vi "pco.labview_Live_Example_COL.vi"() -> ()   [LabVIEW 2019]
doc: "A short program to demonstrate the fundamentals of control and image acquision with the pco.camera series. The program records a sequence of images, with \"live\" updating, until the \"StopRecording\" button is pressed. Use ctrl-H for more help on the individual controls and indicators.\n\nCopyright 2004, 2010 The Cooke Corporation."
uses:
  pco.sdk/CameraAccess/CameraAccess.lvlib
  pco.sdk/ImageSensor/ImageSensor.lvlib
  pco.sdk/TimingControl/TimingControl.lvlib
  pco.recorder/Recorder.lvlib
  pco.sdk/RecordingControl/RecordingControl.lvlib
  pco.sdk/CameraDescription/CameraDescription.lvlib
  pco.convert/Convert.lvlib
  pco.sdk/GeneralCameraControl/GeneralCameraControl.lvlib
  <vilib>/picture/picture.llb/Draw True-Color Pixmap.vi
panel:
  in  "Auto Range Crop":bool
  in  "Auto Range Peak":bool
  out "yHWOffset":u16
  out "xHWOffset":u16
  in  "iContrast [%]":i32 min=-100 max=100 step=1
  in  "Gamma":dbl=1.0 min=0.009999999776482582 max=10.0 step=0.009999999776482582 format="%.2f"
  out "wImgBuf":u16[][](array[numeric])
  in  "whiteBalance":bool
  in  "Zoom [%]":i32(slide)=26 min=10 max=200 step=5 scale=10.0..200.0
  in  "iScale_max":i32=60000 min=0 max=65535 step=1
  in  "iScale_min":i32=200 min=0 max=65535 step=1
  out "colorPattern":u16
  out "phConv":u64
  out "Image":picture
  out "Recorded Images":u32
  in  "TriggerMode":u16(ring) items=["auto sequence"=0, "software trigger"=1, "external exposure start & software trigger"=2, "external exposure control"=3, "external synchronized"=4, "fast external exposure control"=5, "external CDS control"=6, "slow external exposure control"=7, "external synchronized HDSDI"=258]
  in  "Quit":bool
  out "Error":errorcluster {"code" format="%x"}
  in  "Stop Record":bool
  out "Recording On":bool
  in  "roiY1":u16=2 min=2 max=1440 step=1
  in  "roiX1":u16=2 min=2 max=1920 step=1
  in  "roiY0":u16=1 min=1 max=1439 step=1
  in  "roiX0":u16=1 min=1 max=1919 step=1
  out "Image Height":u16
  out "Image Width":u16
  in  "Image Index":u32 max=9
  in  "dwImgCount":u32=10 caption="Required Number of Images" min=4 max=2247
  in  "DelayTimeBase":u16(ring)=2 items=["nanoseconds", "microseconds", "milliseconds"]
  in  "ExposureTimeBase":u16(ring)=2 items=["nanoseconds", "microseconds", "milliseconds"]
  in  "Exposure":u32=10 min=1
  in  "Delay":u32
  in  "Rate":i32(ring) items=["Low", "High"]
  # "This example is only suitable for color cameras\n\nThis example is similar to pco.labview_Live_Example.vi, but suited for color cameras.\nBecause n addition here also the convert library is used in order to get a truecolor image that is displayed\nWith the White Balance button it is possible to set the white balance, \nthe image value range can be selected with iScale_min/iScale_max, additionally contrast and gamma values can be selected\n\nUsage:\nSelect your required image count and the camera setup before you start the program.\nOnce started, the camera will be opened, the recorder will be created, initialized and images will be recorded and displayed automatically\nYou can stop the images by pressing stop record.\nAfter stopped, the image at the selected index will be read out\nTo finish the program click on quit application, this will force free and delete of the recorder and a close camera\nYou can change your required ROI, the value range, scaling, gamma, contrast  and the white balance after and also during record."
  # "pco.labview"
  # "Camera Setup"
  # "Recording Control"
  # "Parameters for image readout"
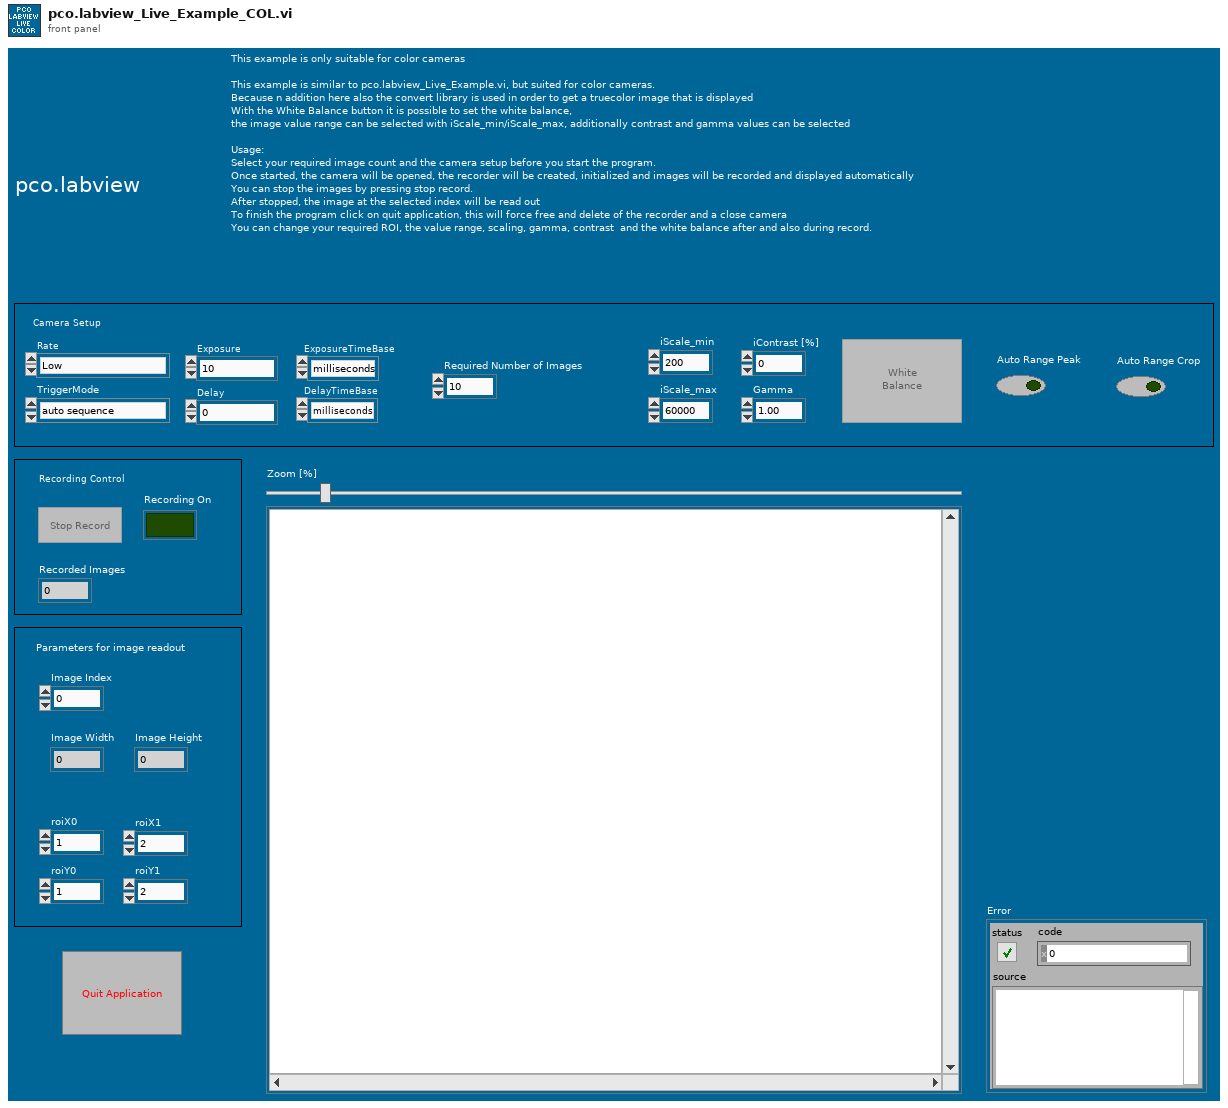
[diagram p1: front panel]
types:
  T1 = enum8{"Enabled", "Disabled", "Disabled and Grayed Out"}
  T2 = cluster{"wSensorTypeDESC":u16, "wSensorSubTypeDESC":u16, "wMaxHorzResStdDESC":u16, "wMaxVertResStdDESC":u16, "wMaxHorzResExtDESC":u16, "wMaxVertResExtDESC":u16, "wDynResDESC":u16, "wMaxBinHorzDESC":u16, "wBinHorzSteppingDESC":u16, "wMaxBinVertDESC":u16, "wBinVertSteppingDESC":u16, "wRoiHorStepsDESC":u16, "wRoiVertStepsDESC":u16, "wNumADCsDESC":u16, "wMinSizeHorzDESC":u16, "dwPixelRateDESC":u32[], "wConvFactDESC":u16[], "sCoolingSetpoints":i16[], "wSoftRoiHorStepsDESC":u16, "wSoftRoiVertStepsDESC":u16, "wIRDESC":u16, "wMinSizeVertDESC":u16, "dwMinDelayDESC":u32, "dwMaxDelayDESC":u32, "dwMinDelayStepDESC":u32, "dwMinExposureDESC":u32, "dwMaxExposureDESC":u32, "dwMinExposureStepDESC":u32, "dwMinDelayIRDESC":u32, "dwMaxDelayIRDESC":u32, "dwMinExposureIRDESC":u32, "dwMaxExposureIRDESC":u32, "wTimeTableDESC":u16, "wDoubleImageDESC":u16, "sMinCoolSetDESC":i16, "sMaxCoolSetDESC":i16, "sDefaultCoolSetDESC":i16, "wPowerDownModeDESC":u16, "wOffsetRegulationDESC":u16, "wColorPatternDESC":u16, "wPatternTypeDESC":u16, "wNumCoolingSetpoints":u16, "dwGeneralCapsDESC1":u32, "dwGeneralCapsDESC2":u32, "dwExtSyncFrequency":u32[], "dwGeneralCapsDESC3":u32, "dwGeneralCapsDESC4":u32}
  T3 = cluster{"wScale_minmax":u16, "iScale_maxmax":i32, "iScale_min":i32, "iScale_max":i32, "iColor_temp":i32, "iColor_tint":i32, "iColor_saturation":i32, "iColor_vibrance":i32, "iContrast":i32, "iGamma":i32, "iSRGB":i32, "pHistogramData":u64, "dwProcessingFlags":u32, "wProzValue4Min":u16, "wProzValue4Max":u16}
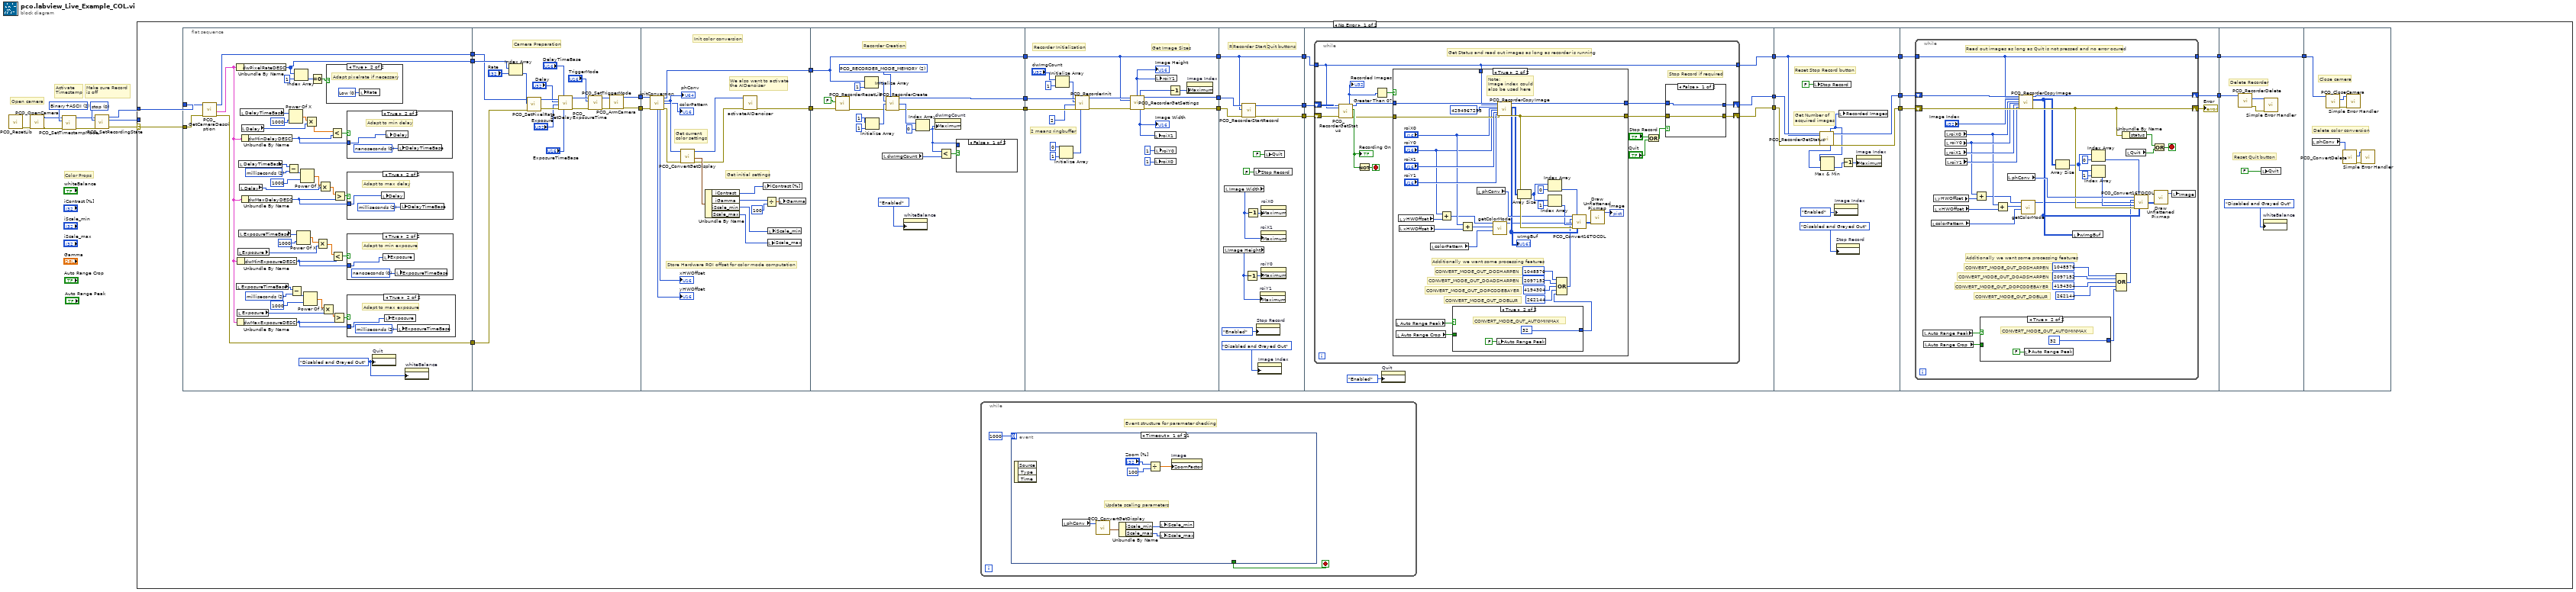
[diagram p0: block diagram]
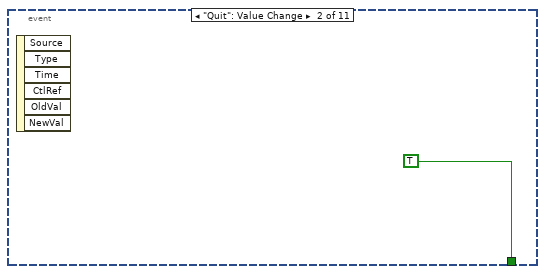
[diagram p2: hidden frame]
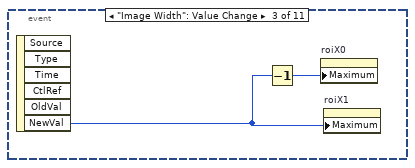
[diagram p3: hidden frame]
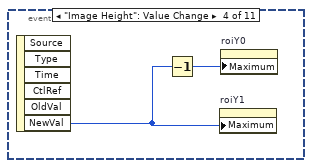
[diagram p4: hidden frame]
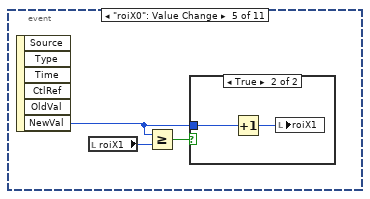
[diagram p5: hidden frame]
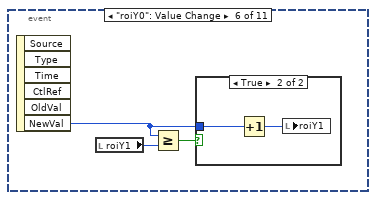
[diagram p7: hidden frame]
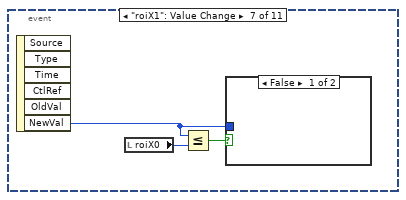
[diagram p9: hidden frame]
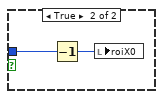
[diagram p10: hidden frame]
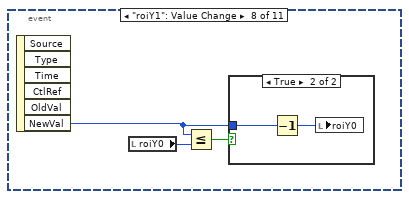
[diagram p11: hidden frame]
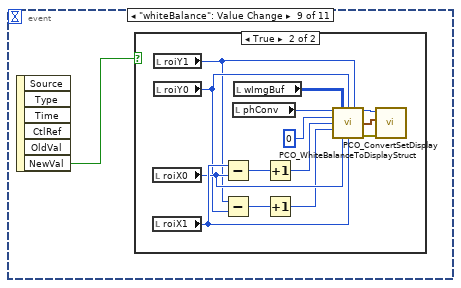
[diagram p13: hidden frame]
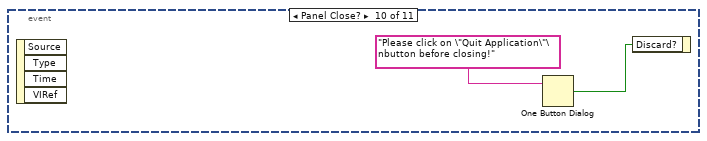
[diagram p15: hidden frame]
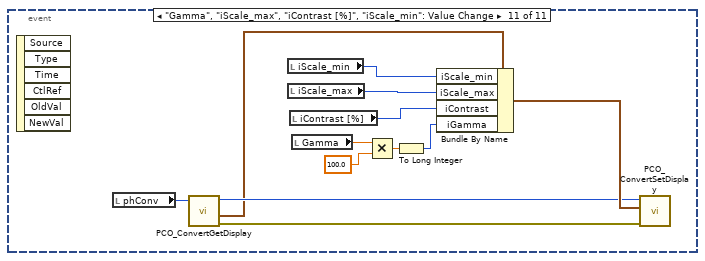
[diagram p16: hidden frame]
diagram:
  w5 = u16 2 items=["OFF", "Binary", "Binary+ASCII", "ASCII"] ("wTimeStampMode")
  w9 = u16 0 items=["stop", "run"] ("wRecState")
  # "Color Props"
  # "Activate\nTimestamp"
  # "Make sure Record \nis off"
  # "Open camera"
  n1 = call "PCO_ResetLib.vi"() -> ("error out"=w10:errorcluster)  [unwired: 10 in, 1 out]
  n2 = call "PCO_OpenCamera.vi"("error in (no error)"=w10) -> ("error out"=w3:errorcluster, "ph out"=w4:u64)  [unwired: 8 in, 1 out]
  n3 = call "PCO_SetTimestampMode.vi"("error in (no error)"=w3, "wTimeStampMode"=w5, "ph"=w4) -> ("error out"=w2:errorcluster, "ph out"=w1:u64)  [unwired: 6 in, 1 out]
  n4 = call "PCO_SetRecordingState.vi"("error in (no error)"=w2, "wRecState"=w9, "ph"=w1) -> ("error out"=w7:errorcluster, "ErrorMessage"=w6:i32, "ph out"=w8:u64)  [unwired: 6 in]
  n5 = case shown="No Error" w7 {
    selector: w7 -> [w36 w385]
    tunnel: w8 -> [w37 _]
    tunnel: w6 -> [_ w384]
    frame No Error {
      n6 = flat-sequence {
        tunnel: w36 -> [w139]
        tunnel: w37 -> [w140]
        tunnel: [w135] -> w20
        tunnel: [w142] -> w19
        tunnel: [w141] -> w18
        tunnel: [w154] -> w14
        tunnel: [w155] -> w12
        tunnel: w20 -> [w158]
        tunnel: w19 -> [w152]
        tunnel: w18 -> [w153]
        tunnel: w14 -> [w178]
        tunnel: [w174] -> w13
        tunnel: w12 -> [w179]
        tunnel: [w173] -> w11
        tunnel: w13 -> [w204]
        tunnel: w11 -> [w193]
        tunnel: [w195] -> w35
        tunnel: [w194] -> w34
        tunnel: [w193] -> w31
        tunnel: w35 -> [w226]
        tunnel: w34 -> [w225]
        tunnel: [w216] -> w33
        tunnel: [w217] -> w32
        tunnel: w31 -> [w215]
        tunnel: [w215] -> w30
        tunnel: w33 -> [w237]
        tunnel: w32 -> [w229]
        tunnel: w30 -> [w236]
        tunnel: [w236] -> w17
        tunnel: [w231] -> w16
        tunnel: [w230] -> w15
        tunnel: w17 -> [w246]
        tunnel: [w245] -> w28
        tunnel: [w244] -> w26
        tunnel: [w243] -> w24
        tunnel: w16 -> [w241]
        tunnel: w15 -> [w240]
        tunnel: [w317] -> w29
        tunnel: w28 -> [w319]
        tunnel: [w316] -> w27
        tunnel: w26 -> [w320]
        tunnel: [w318] -> w25
        tunnel: w24 -> [w318]
        tunnel: w29 -> [w328]
        tunnel: w27 -> [w327]
        tunnel: w25 -> [w326]
        tunnel: [w324] -> w23
        tunnel: [w323] -> w22
        tunnel: w23 -> [w376]
        tunnel: w22 -> [w373]
        tunnel: [w373] -> w21
        tunnel: w21 -> [w383]
        frame #0 {
          w101 = u16 2 items=["nanoseconds", "microseconds", "milliseconds"] ("DelayTimeBase")
          w102 = u16 2 items=["nanoseconds", "microseconds", "milliseconds"] ("DelayTimeBase")
          w134 = T1."Disabled and Grayed Out" ("Disabled")
          n7 = call "PCO_GetCameraDescription.vi"("error in (no error)"=w139, "ph"=w140) -> ("error out"=w142:errorcluster, "strDescription"=w103:T2, "ph out"=w141:u64)  [unwired: 6 in, 1 out]
          n8 = Unbundle By Name(w103) -> ("dwPixelRateDESC"=w135:u32[])
          n9 = local read "ExposureTimeBase"() -> (w110:u16)
          n10 = Unbundle By Name(w103) -> ("dwMaxExposureDESC"=w132:u32)
          n11 = Unbundle By Name(w103) -> ("dwMinExposureDESC"=w131:u32)
          n12 = local read "Exposure"() -> (w116:u32)
          n13 = local read "Exposure"() -> (w114:u32)
          n14 = local read "DelayTimeBase"() -> (w111:u16)
          n15 = local read "ExposureTimeBase"() -> (w126:u16)
          n16 = local read "Delay"() -> (w120:u32)
          n17 = local read "DelayTimeBase"() -> (w130:u16)
          n18 = local read "Delay"() -> (w128:u32)
          n19 = Unbundle By Name(w103) -> ("dwMinDelayDESC"=w104:u32)
          n20 = Unbundle By Name(w103) -> ("dwMaxDelayDESC"=w133:u32)
          n21 = Subtract(x=w111, y=w102) -> (x-y=w123:i32)
          n22 = Power Of X(1:u32 1000 ("Delay"), 2:w130) -> (0:w129:dbl)
          n23 = Subtract(x=w110, y=w101) -> (x-y=w117:i32)
          n24 = Index Array(array=w135, index=1) -> (element=w137:u32)
          n25 = Power Of X(1:u32 1000 ("Delay"), 2:w126) -> (0:w125:dbl)
          n26 = Power Of X(1:u32 1000 ("Delay"), 2:w123) -> (0:w121:dbl)
          n27 = Power Of X(1:u32 1000 ("Delay"), 2:w117) -> (0:w118:dbl)
          n28 = Multiply(x=w129, y=w128) -> (x*y=w127:dbl)
          n29 = Equal To 0?(x=w137) -> (x = 0?=w136:bool)
          n30 = Multiply(x=w125, y=w114) -> (x*y=w113:dbl)
          n31 = Multiply(x=w121, y=w120) -> (x*y=w122:dbl)
          n32 = Multiply(x=w118, y=w116) -> (x*y=w115:dbl)
          n33 = case shown="True" w136 {
            frame False {
            }
            frame True {
              w151 = 0 items=["Low", "High"] ("Rate")
              # "Adapt pixelrate if necessary"
              n34 = local write "Rate"(w151) -> ()
            }
          }
          n35 = Less?(x=w127, y=w104) -> (x < y?=w105:bool)
          n36 = Less?(x=w113, y=w131) -> (x < y?=w112:bool)
          n37 = Greater?(x=w115, y=w132) -> (0:w119:bool)
          n38 = Greater?(x=w122, y=w133) -> (0:w124:bool)
          n39 = case shown="True" w105 {
            tunnel: w104 -> [_ w144]
            frame False {
            }
            frame True {
              w143 = u16 0 items=["nanoseconds", "microseconds", "milliseconds"] ("DelayTimeBase")
              # "Adapt to min delay"
              n40 = local write "Delay"(w144) -> ()
              n41 = local write "DelayTimeBase"(w143) -> ()
            }
          }
          n42 = case shown="True" w124 {
            tunnel: w133 -> [_ w150]
            frame False {
            }
            frame True {
              w149 = u16 2 items=["nanoseconds", "microseconds", "milliseconds"] ("DelayTimeBase")
              # "Adapt to max delay"
              n43 = local write "Delay"(w150) -> ()
              n44 = local write "DelayTimeBase"(w149) -> ()
            }
          }
          n45 = case shown="True" w112 {
            tunnel: w131 -> [_ w148]
            frame False {
            }
            frame True {
              w147 = u16 0 items=["nanoseconds", "microseconds", "milliseconds"] ("DelayTimeBase")
              # "Adapt to min exposure"
              n46 = local write "Exposure"(w148) -> ()
              n47 = local write "ExposureTimeBase"(w147) -> ()
            }
          }
          n48 = case shown="True" w119 {
            tunnel: w132 -> [_ w146]
            frame False {
            }
            frame True {
              w145 = u16 2 items=["nanoseconds", "microseconds", "milliseconds"] ("DelayTimeBase")
              # "Adapt to max exposure"
              n49 = local write "Exposure"(w146) -> ()
              n50 = local write "ExposureTimeBase"(w145) -> ()
            }
          }
          n51 = property on="Quit" class="Bool (strict)"("DisabledEnum"=w134) -> ()  [unwired: 2 in, 2 out]
          n52 = property on="whiteBalance" class="Bool (strict)"("DisabledEnum"=w134) -> ()  [unwired: 2 in, 2 out]
        }
        frame #1 {
          # "Camera Preparation"
          n53 = Index Array(array=w158, index="Rate") -> (element=w168:u32)
          n54 = call "PCO_SetPixelRate.vi"("error in (no error)"=w152, "dwPixelRate"=w168, "ph"=w153) -> ("error out"=w166:errorcluster, "ph out"=w167:u64)  [unwired: 6 in, 1 out]
          n55 = call "PCO_SetDelayExposureTime.vi"("wTimeBaseExposure"="ExposureTimeBase", "wTimeBaseDelay"="DelayTimeBase", "error in (no error)"=w166, "dwExposure"="Exposure", "dwDelay"="Delay", "ph"=w167) -> ("error out"=w160:errorcluster, "ph out"=w161:u64)  [unwired: 3 in, 1 out]
          n56 = call "PCO_SetTriggerMode.vi"("error in (no error)"=w160, "wTriggerMode"="TriggerMode", "ph"=w161) -> ("error out"=w156:errorcluster, "ph out"=w157:u64)  [unwired: 6 in, 1 out]
          n57 = call "PCO_ArmCamera.vi"("error in (no error)"=w156, "ph"=w157) -> ("error out"=w154:errorcluster, "ph out"=w155:u64)  [unwired: 7 in, 1 out]
        }
        frame #2 {
          # "We also want to activate\nthe AIDenoiser"
          # "Init color conversion"
          # "Get current\ncolor settings"
          # "Store Hardware ROI offset for color mode computation"
          # "Get initial settings"
          n58 = call "initConversion.vi"("phCam"=w179, "error in (no error)"=w178) -> ("ph out"=w173:u64, "phConv"=w181:u64, "colorPattern"=→"colorPattern":u16, "yOffset"=→"yHWOffset":u16, "xOffset"=→"xHWOffset":u16, "error out"=w182:errorcluster)  [unwired: 8 in]
          "phConv" <- w181
          n59 = call "PCO_ConvertGetDisplay.vi"("error in (no error)"=w182, "ph"=w181) -> ("error out"=w176:errorcluster, "strDisplay"=w177:T3, "ph out"=w175:u64)  [unwired: 6 in, 1 out]
          n60 = Unbundle By Name(w177) -> ("iContrast"=w185:i32, "iGamma"=w172:i32, "iScale_min"=w186:i32, "iScale_max"=w187:i32)
          n61 = call "activateAIDenoiser.vi"("phConv in"=w175, "error in (no error)"=w176) -> ("error out"=w174:errorcluster)  [unwired: 12 in, 1 out]
          n62 = local write "iContrast [%]"(w185) -> ()
          n63 = Divide(x=w172, y=100) -> (x/y=w170:dbl)
          n64 = local write "iScale_max"(w187) -> ()
          n65 = local write "iScale_min"(w186) -> ()
          n66 = local write "Gamma"(w170) -> ()
        }
        frame #3 {
          w188 = u16 2 items=["PCO_RECORDER_MODE_FILE"=1, "PCO_RECORDER_MODE_MEMORY"=2, "PCO_RECORDER_MODE_CAMRAM"=3] ("dwRecMode")
          # "Recorder Creation"
          n67 = call "PCO_RecorderResetLib.vi"("error in (no error)"=w204, "bSilent"=FALSE) -> ("error out"=w196:errorcluster)  [unwired: 8 in, 1 out]
          n68 = Initialize Array(w193, 1 ("dimension size")) -> (w202:u64[])
          n69 = Initialize Array(u32 1 ("dimension size"), 1 ("dimension size")) -> (w199:u32[])
          n70 = local read "dwImgCount"() -> (w190:u32)
          n71 = call "PCO_RecorderCreate.vi"("wRecMode"=w188, "phCamArr"=w202, "dwImgDistributionArr"=w199, "error in (no error)"=w196) -> ("phRec out"=w194:u64, "dwMaxImgCountArr"=w198:u32[], "error out"=w195:errorcluster)  [unwired: 8 in, 1 out]
          n72 = property on="whiteBalance" class="Bool (strict)"("DisabledEnum"=T1."Enabled" ("Disabled")) -> ()  [unwired: 2 in, 2 out]
          n73 = Index Array(array=w198, index=0) -> (element=w191:u32)
          n74 = property on="dwImgCount" class="DigNum (strict)"("Maximum"=w191) -> ()  [unwired: 2 in, 2 out]
          n75 = Less?(x=w191, y=w190) -> (x < y?=w192:bool)
          n76 = case shown="False" w192 {
            tunnel: w191 -> [_ w206]
            frame False {
            }
            frame True {
              n77 = local write "dwImgCount"(w206) -> ()
            }
          }
        }
        frame #4 {
          # "2 means ringbuffer"
          # "Get Image Sizes"
          # "Recorder Initialization"
          n78 = Initialize Array("dwImgCount", 1 ("dimension size")) -> (w222:u32[])
          n79 = Initialize Array(u16 0 ("element"), 1 ("dimension size")) -> (w207:u16[])
          n80 = call "PCO_RecorderInit.vi"("wRamSegmentArr"=w207, "error in (no error)"=w226, "wType"=u16 2, "dwImgCountArr"=w222, "phRec"=w225) -> ("error out"=w221:errorcluster, "phRec out"=w220:u64)  [unwired: 4 in, 1 out]
          n81 = call "PCO_RecorderGetSettings.vi"("phRec"=w220, "phCam"=w215, "error in (no error)"=w221) -> ("wHeight"=w214:u16, "dwReqImgCount"=w211:u32, "phRec out"=w216:u64, "wWidth"=w213:u16, "error out"=w217:errorcluster)  [unwired: 4 in, 4 out]
          "Image Height" <- w214
          "Image Width" <- w213
          n82 = local write "roiX1"(w213) -> ()
          n83 = local write "roiX0"(u16 1 ("roiY0")) -> ()
          n84 = local write "roiY0"(u16 1 ("roiY0")) -> ()
          n85 = local write "roiY1"(w214) -> ()
          n86 = Decrement(x=w211) -> (x-1=w212:u32)
          n87 = property on="Image Index" class="DigNum (strict)"("Maximum"=w212) -> ()  [unwired: 2 in, 2 out]
        }
        frame #5 {
          # "Reset Stop and Quit buttons"
          # "Recorder Start"
          n88 = local read "Image Height"() -> (w233:u16)
          n89 = local read "Image Width"() -> (w232:u16)
          n90 = call "PCO_RecorderStartRecord.vi"("error in (no error)"=w229, "phCam"=w236, "phRec"=w237) -> ("error out"=w230:errorcluster, "phRec out"=w231:u64)  [unwired: 6 in, 1 out]
          n91 = Decrement(x=w233) -> (x-1=w234:u16)
          n92 = Decrement(x=w232) -> (x-1=w235:u16)
          n93 = local write "Stop Record"(FALSE ("Stop Record")) -> ()
          n94 = property on="Stop Record" class="Bool (strict)"("DisabledEnum"=T1."Enabled" ("Disabled")) -> ()  [unwired: 2 in, 2 out]
          n95 = property on="Image Index" class="DigNum (strict)"("DisabledEnum"=T1."Disabled and Grayed Out" ("Disabled")) -> ()  [unwired: 2 in, 2 out]
          n96 = property on="roiY1" class="DigNum (strict)"("Maximum"=w233) -> ()  [unwired: 2 in, 2 out]
          n97 = property on="roiX1" class="DigNum (strict)"("Maximum"=w232) -> ()  [unwired: 2 in, 2 out]
          n98 = property on="roiY0" class="DigNum (strict)"("Maximum"=w234) -> ()  [unwired: 2 in, 2 out]
          n99 = property on="roiX0" class="DigNum (strict)"("Maximum"=w235) -> ()  [unwired: 2 in, 2 out]
          n100 = local write "Quit"(FALSE ("Stop")) -> ()
        }
        frame #6 {
          n101 = while {
            tunnel: w246 -> [w250]
            shift-right: [w254] -> w244
            shift-left: w240 -> [w262]
            shift-right: [w255] -> w245
            shift-left: w241 -> [w258]
            tunnel: [w250] -> w243
            stop <- w257 stop-if-true
            # "Stop Record if required"
            # "Get Status and read out images as long as recorder is running"
            n102 = call "PCO_RecorderGetStatus.vi"("phRec"=w258, "phCam"=w250, "error in (no error)"=w262) -> ("dwProcImgCount"=w247:u32, "phRec out"=w260:u64, "bIsRunning"=w261:bool, "error out"=w259:errorcluster)  [unwired: 5 in, 8 out]
            "Recording On" <- w261
            "Recorded Images" <- w247
            n103 = Not(x=w261) -> (.not. x?=w257:bool)
            n104 = Greater Than 0?(x=w247) -> (x > 0?=w248:bool)
            n105 = case shown="True" w248 {
              tunnel: w260 -> [w264 w297]
              tunnel: w259 -> [w263 w293]
              tunnel: [w264 w292] -> w251
              tunnel: w250 -> [_ w290]
              tunnel: [w263 w288] -> w249
              frame False {
              }
              frame True {
                # "CONVERT_MODE_OUT_DOBLUR"
                # "CONVERT_MODE_OUT_DOPCODEBAYER"
                # "CONVERT_MODE_OUT_DOADSHARPEN"
                # "CONVERT_MODE_OUT_DOSHARPEN"
                # "Additionally we want some processing features"
                # "Note: \nImage index could \nalso be used here"
                n106 = local read "Auto Range Peak"() -> (w267:bool)
                n107 = local read "Auto Range Crop"() -> (w266:bool)
                n108 = local read "yHWOffset"() -> (w270:u16)
                n109 = local read "xHWOffset"() -> (w272:u16)
                n110 = local read "colorPattern"() -> (w280:u16)
                n111 = Add(x="roiY0", y=w270) -> (x+y=w268:u16)
                n112 = case shown="True" w267 {
                  tunnel: [w298 32 ("colorMode")] -> w265
                  tunnel: w266 -> [w299 _]
                  frame False {
                    n113 = case shown="True" w299 {
                      tunnel: [0 ("colorMode") 64 ("colorMode")] -> w298
                      frame False {
                      }
                      frame True {
                        # "CONVERT_MODE_OUT_AUTOMINMAX_SM"
                        n114 = local write "Auto Range Crop"(FALSE ("Auto Range Crop")) -> ()
                      }
                    }
                  }
                  frame True {
                    # "CONVERT_MODE_OUT_AUTOMINMAX"
                    n115 = local write "Auto Range Peak"(FALSE ("Auto Range Peak")) -> ()
                  }
                }
                n116 = Add(x="roiX0", y=w272) -> (x+y=w273:u16)
                n117 = local read "phConv"() -> (w287:u64)
                n118 = call "getColorMode.vi"("wColorPatternDESC"=w280, "wRoiX0"=w273, "wRoiY0"=w268) -> ("colorMode"=w275:i32)  [unwired: 8 in]
                n119 = call "PCO_RecorderCopyImage.vi"("phRec"=w297, "phCam"=w290, "dwImgIdx"=u32 4294967295, "wRoiX0"="roiX0", "wRoiY0"="roiY0", "wRoiX1"="roiX1", "wRoiY1"="roiY1", "error in (no error)"=w293) -> ("phRec out"=w292:u64, "wImgBuf"=w286:u16[][], "error out"=w288:errorcluster)  [unwired: 13 in, 4 out]
                "wImgBuf" <- w286
                n120 = Array Size(array=w286) -> (size(s)=w282:i32[])
                n121 = Index Array(array=w282, index=0) -> (element=w284:i32)
                n122 = Index Array(array=w282, index=1) -> (element=w281:i32)
                n123 = Compound Arithmetic op=OR ("Mehrfacharithmetik")(1048576 ("colorMode"), 2097152 ("colorMode"), 4194304 ("colorMode"), 262144 ("colorMode"), w265) -> (w274:i32)
                n124 = call "PCO_Convert16TOCOL.vi"("ph"=w287, "height"=w284, "mode"=w274, "icolmode"=w275, "width"=w281, "error in (no error)"=w288, "b16"=w286) -> ("b32"=w289:u32[][])  [unwired: 5 in, 3 out]
                n125 = call-poly <vilib>:"Draw Unflattened Pixmap.vi"("data (RGB format)"=w289) -> ("new picture"=→"Image":picture)  [unwired: 8 in]
              }
            }
            n126 = Or(x="Stop Record", y="Quit") -> (x .or. y?=w256:bool)
            n127 = case shown="False" w256 {
              tunnel: w251 -> [w306 w310]
              tunnel: w249 -> [w305 w309]
              tunnel: [w306 w307] -> w255
              tunnel: [w305 w308] -> w254
              frame False {
              }
              frame True {
                n128 = call "PCO_RecorderStopRecord.vi"("error in (no error)"=w309, "phRec"=w310) -> ("error out"=w308:errorcluster, "phRec out"=w307:u64)  [unwired: 7 in, 1 out]
              }
            }
          }
          n129 = property on="Quit" class="Bool (strict)"("DisabledEnum"=T1."Enabled" ("Disabled")) -> ()  [unwired: 2 in, 2 out]
        }
        frame #7 {
          # "Get Number of \nacquired images"
          # "Reset Stop Record button"
          n130 = local write "Stop Record"(FALSE ("Stop Record")) -> ()
          n131 = call "PCO_RecorderGetStatus.vi"("phRec"=w319, "phCam"=w318, "error in (no error)"=w320) -> ("dwProcImgCount"=w315:u32, "dwReqImgCount"=w313:u32, "phRec out"=w317:u64, "error out"=w316:errorcluster)  [unwired: 5 in, 8 out]
          n132 = Max & Min(x=w315, y=w313) -> (min(x,y)=w314:u32)  [unwired: 1 out]
          n133 = property on="Image Index" class="DigNum (strict)"("DisabledEnum"=T1."Enabled" ("Disabled")) -> ()  [unwired: 2 in, 2 out]
          n134 = property on="Stop Record" class="Bool (strict)"("DisabledEnum"=T1."Disabled and Grayed Out" ("Disabled")) -> ()  [unwired: 2 in, 2 out]
          n135 = local write "Recorded Images"(w315) -> ()
          n136 = Decrement(x=w314) -> (x-1=w321:u32)
          n137 = property on="Image Index" class="DigNum (strict)"("Maximum"=w321) -> ()  [unwired: 2 in, 2 out]
        }
        frame #8 {
          n138 = while {
            shift-right: [w351] -> w325
            shift-left: w327 -> [w361]
            shift-right: [w355] -> w324
            shift-left: w328 -> [w360]
            tunnel: w326 -> [w354]
            tunnel: [w354] -> w323
            stop <- w362 stop-if-true
            # "CONVERT_MODE_OUT_DOBLUR"
            # "CONVERT_MODE_OUT_DOPCODEBAYER"
            # "CONVERT_MODE_OUT_DOADSHARPEN"
            # "CONVERT_MODE_OUT_DOSHARPEN"
            # "Additionally we want some processing features"
            # "Read out images as long as Quit is not pressed and no error ocured"
            n139 = local read "Auto Range Peak"() -> (w330:bool)
            n140 = local read "Auto Range Crop"() -> (w331:bool)
            n141 = local read "colorPattern"() -> (w345:u16)
            n142 = local read "yHWOffset"() -> (w337:u16)
            n143 = local read "xHWOffset"() -> (w336:u16)
            n144 = local read "roiX0"() -> (w334:u16)
            n145 = local read "roiX1"() -> (w358:u16)
            n146 = local read "roiY0"() -> (w335:u16)
            n147 = local read "roiY1"() -> (w357:u16)
            n148 = Add(x=w335, y=w337) -> (x+y=w332:u16)
            n149 = case shown="True" w330 {
              tunnel: [w365 32 ("colorMode")] -> w329
              tunnel: w331 -> [w366 _]
              frame False {
                n150 = case shown="True" w366 {
                  tunnel: [0 ("colorMode") 64 ("colorMode")] -> w365
                  frame False {
                  }
                  frame True {
                    # "CONVERT_MODE_OUT_AUTOMINMAX_SM"
                    n151 = local write "Auto Range Crop"(FALSE ("Auto Range Crop")) -> ()
                  }
                }
              }
              frame True {
                # "CONVERT_MODE_OUT_AUTOMINMAX"
                n152 = local write "Auto Range Peak"(FALSE ("Auto Range Peak")) -> ()
              }
            }
            n153 = Add(x=w334, y=w336) -> (x+y=w333:u16)
            n154 = local read "phConv"() -> (w353:u64)
            n155 = call "PCO_RecorderCopyImage.vi"("phRec"=w360, "phCam"=w354, "dwImgIdx"="Image Index", "wRoiX0"=w334, "wRoiY0"=w335, "wRoiX1"=w358, "wRoiY1"=w357, "error in (no error)"=w361) -> ("phRec out"=w355:u64, "wImgBuf"=w344:u16[][], "error out"=w351:errorcluster)  [unwired: 13 in, 4 out]
            n156 = call "getColorMode.vi"("wColorPatternDESC"=w345, "wRoiX0"=w333, "wRoiY0"=w332) -> ("colorMode"=w339:i32)  [unwired: 8 in]
            n157 = Array Size(array=w344) -> (size(s)=w348:i32[])
            n158 = local write "wImgBuf"(w344) -> ()
            n159 = Index Array(array=w348, index=0) -> (element=w347:i32)
            n160 = Index Array(array=w348, index=1) -> (element=w346:i32)
            n161 = Compound Arithmetic op=OR ("Mehrfacharithmetik")(1048576 ("colorMode"), 2097152 ("colorMode"), 4194304 ("colorMode"), 262144 ("colorMode"), w329) -> (w338:i32)
            n162 = Unbundle By Name(w351) -> ("status"=w364:bool)
            n163 = local read "Quit"() -> (w363:bool)
            n164 = call "PCO_Convert16TOCOL.vi"("ph"=w353, "height"=w347, "mode"=w338, "icolmode"=w339, "width"=w346, "error in (no error)"=w351, "b16"=w344) -> ("b32"=w352:u32[][])  [unwired: 5 in, 3 out]
            n165 = Or(x=w364, y=w363) -> (x .or. y?=w362:bool)
            n166 = call-poly <vilib>:"Draw Unflattened Pixmap.vi"("data (RGB format)"=w352) -> ("new picture"=w356:picture)  [unwired: 8 in]
            n167 = local write "Image"(w356) -> ()
          }
          "Error" <- w325
        }
        frame #9 {
          # "Delete Recorder"
          # "Reset Quit button"
          n168 = call "PCO_RecorderDelete.vi"("phRec"=w376) -> ("error out"=w374:errorcluster, "ErrorMessage"=w375:i32)  [unwired: 9 in]
          n169 = local write "Quit"(FALSE ("Stop Record")) -> ()
          n170 = property on="whiteBalance" class="Bool (strict)"("DisabledEnum"=T1."Disabled and Grayed Out" ("Disabled")) -> ()  [unwired: 2 in, 2 out]
          n171 = call <vilib>:"Simple Error Handler.vi"("error code (no error:0)"=w375, "error in (no error)"=w374) -> ()  [unwired: 3 in, 5 out]
        }
        frame #10 {
          # "Delete color conversion"
          # "Close camera"
          n172 = local read "phConv"() -> (w380:u64)
          n173 = call "PCO_CloseCamera.vi"("ph"=w383) -> ("error out"=w381:errorcluster, "ErrorMessage"=w382:i32)  [unwired: 9 in]
          n174 = call "PCO_ConvertDelete.vi"("ph"=w380) -> ("error out"=w378:errorcluster, "ErrorMessage"=w379:i32)  [unwired: 9 in]
          n175 = call <vilib>:"Simple Error Handler.vi"("error code (no error:0)"=w382, "error in (no error)"=w381) -> ()  [unwired: 3 in, 5 out]
          n176 = call <vilib>:"Simple Error Handler.vi"("error code (no error:0)"=w379, "error in (no error)"=w378) -> ()  [unwired: 3 in, 5 out]
        }
      }
      n177 = while {
        stop <- w39 stop-if-true
        # "Event structure for parameter checking"
        n178 = event shown="[0] Timeout" {
          selector: _ -> [_ _ _ _ _ _ _ _ _ _ _]
          dyn-events: _ -> [_ _ _ _ _ _ _ _ _ _ _]
          timeout: 1000 -> [_ _ _ _ _ _ _ _ _ _ _]
          tunnel: [_ TRUE _ _ _ _ _ _ _ _ _] -> w39
          event Timeout {
            # "Update scaling parameters"
            n179 = event-data() -> ()  [unwired: 1 in, 3 out]
            n180 = local read "phConv"() -> (w43:u64)
            n181 = call "PCO_ConvertGetDisplay.vi"("ph"=w43) -> ("strDisplay"=w42:T3)  [unwired: 7 in, 3 out]
            n182 = Unbundle By Name(w42) -> ("iScale_min"=w41:i32, "iScale_max"=w40:i32)
            n183 = Divide(x="Zoom [%]", y=100) -> (x/y=w44:dbl)
            n184 = local write "iScale_min"(w41) -> ()
            n185 = local write "iScale_max"(w40) -> ()
            n186 = property on="Image" class="Pict"("ZoomFactor"=w44) -> ()  [unwired: 2 in, 2 out]
          }
          event "Quit": Value Change {
            n187 = event-data() -> ()  [unwired: 1 in, 6 out]
          }
          event "Image Width": Value Change {
            n188 = event-data() -> ("NewVal"=w48:u16)  [unwired: 1 in, 5 out]
            n189 = Decrement(x=w48) -> (x-1=w49:u16)
            n190 = property on="roiX0" class="DigNum (strict)"("Maximum"=w49) -> ()  [unwired: 2 in, 2 out]
            n191 = property on="roiX1" class="DigNum (strict)"("Maximum"=w48) -> ()  [unwired: 2 in, 2 out]
          }
          event "Image Height": Value Change {
            n192 = event-data() -> ("NewVal"=w50:u16)  [unwired: 1 in, 5 out]
            n193 = Decrement(x=w50) -> (x-1=w51:u16)
            n194 = property on="roiY1" class="DigNum (strict)"("Maximum"=w50) -> ()  [unwired: 2 in, 2 out]
            n195 = property on="roiY0" class="DigNum (strict)"("Maximum"=w51) -> ()  [unwired: 2 in, 2 out]
          }
          event "roiX0": Value Change {
            n196 = event-data() -> ("NewVal"=w52:u16)  [unwired: 1 in, 5 out]
            n197 = local read "roiX1"() -> (w54:u16)
            n198 = Greater Or Equal?(x=w52, y=w54) -> (x >= y?=w53:bool)
            n199 = case shown="True" w53 {
              tunnel: w52 -> [_ w56]
              frame False {
              }
              frame True {
                n200 = Increment(x=w56) -> (x+1=w55:u16)
                n201 = local write "roiX1"(w55) -> ()
              }
            }
          }
          event "roiY0": Value Change {
            n202 = event-data() -> ("NewVal"=w57:u16)  [unwired: 1 in, 5 out]
            n203 = local read "roiY1"() -> (w59:u16)
            n204 = Greater Or Equal?(x=w57, y=w59) -> (x >= y?=w58:bool)
            n205 = case shown="True" w58 {
              tunnel: w57 -> [_ w61]
              frame False {
              }
              frame True {
                n206 = Increment(x=w61) -> (x+1=w60:u16)
                n207 = local write "roiY1"(w60) -> ()
              }
            }
          }
          event "roiX1": Value Change {
            n208 = event-data() -> ("NewVal"=w62:u16)  [unwired: 1 in, 5 out]
            n209 = local read "roiX0"() -> (w64:u16)
            n210 = Less Or Equal?(x=w62, y=w64) -> (x <= y?=w63:bool)
            n211 = case shown="False" w63 {
              tunnel: w62 -> [_ w66]
              frame False {
              }
              frame True {
                n212 = Decrement(x=w66) -> (x-1=w65:u16)
                n213 = local write "roiX0"(w65) -> ()
              }
            }
          }
          event "roiY1": Value Change {
            n214 = event-data() -> ("NewVal"=w67:u16)  [unwired: 1 in, 5 out]
            n215 = local read "roiY0"() -> (w69:u16)
            n216 = Less Or Equal?(x=w67, y=w69) -> (x <= y?=w68:bool)
            n217 = case shown="True" w68 {
              tunnel: w67 -> [_ w71]
              frame False {
              }
              frame True {
                n218 = Decrement(x=w71) -> (x-1=w70:u16)
                n219 = local write "roiY0"(w70) -> ()
              }
            }
          }
          event "whiteBalance": Value Change {
            n220 = event-data() -> ("NewVal"=w72:bool)  [unwired: 1 in, 5 out]
            n221 = case shown="True" w72 {
              frame False {
              }
              frame True {
                n222 = local read "roiX0"() -> (w82:u16)
                n223 = local read "roiX1"() -> (w83:u16)
                n224 = local read "roiY1"() -> (w73:u16)
                n225 = local read "roiY0"() -> (w74:u16)
                n226 = Subtract(x=w83, y=w82) -> (x-y=w81:u16)
                n227 = Subtract(x=w73, y=w74) -> (x-y=w80:u16)
                n228 = local read "phConv"() -> (w85:u64)
                n229 = local read "wImgBuf"() -> (w86:u16[][])
                n230 = Increment(x=w81) -> (x+1=w78:u16)
                n231 = Increment(x=w80) -> (x+1=w79:u16)
                n232 = call "PCO_WhiteBalanceToDisplayStruct.vi"("ph"=w85, "gb12"=w86, "y_min"=w74, "y_max"=w73, "mode"=0, "width"=w78, "height"=w79, "x_min"=w82, "x_max"=w83) -> ("ph out"=w75:u64, "strDisplay"=w76:T3, "error out"=w77:errorcluster)  [unwired: 3 in, 1 out]
                n233 = call "PCO_ConvertSetDisplay.vi"("error in (no error)"=w77, "strDisplay"=w76, "ph"=w75) -> ()  [unwired: 6 in, 3 out]
              }
            }
          }
          event Panel Close? {
            n234 = event-data() -> ()  [unwired: 1 in, 4 out]
            n235 = One Button Dialog(message="Please click on \"Quit Application\"\nbutton before closing!") -> (true=w87:bool)  [unwired: 1 in]
            n236 = event-data("Discard?"=w87) -> ()  [unwired: 1 in, 1 out]
          }
          event "Gamma", "iScale_max", "iContrast [%]", "iScale_min": Value Change {
            n237 = event-data() -> ()  [unwired: 1 in, 6 out]
            n238 = local read "phConv"() -> (w97:u64)
            n239 = call "PCO_ConvertGetDisplay.vi"("ph"=w97) -> ("error out"=w94:errorcluster, "strDisplay"=w93:T3, "ph out"=w95:u64)  [unwired: 7 in, 1 out]
            n240 = local read "iScale_min"() -> (w98:i32)
            n241 = local read "iScale_max"() -> (w99:i32)
            n242 = local read "iContrast [%]"() -> (w100:i32)
            n243 = local read "Gamma"() -> (w92:dbl)
            n244 = Multiply(x=w92, y=100.0) -> (x*y=w90:dbl)
            n245 = To Long Integer(number=w90) -> (32bit integer=w89:i32)
            n246 = Bundle By Name(cluster=w93, "iScale_min"=w98, "iScale_max"=w99, "iContrast"=w100, "iGamma"=w89) -> (w96:T3)
            n247 = call "PCO_ConvertSetDisplay.vi"("error in (no error)"=w94, "strDisplay"=w96, "ph"=w95) -> ()  [unwired: 6 in, 3 out]
          }
        }
      }
    }
    frame Error {
      n248 = call <vilib>:"Simple Error Handler.vi"("error code (no error:0)"=w384, "error in (no error)"=w385) -> ()  [unwired: 3 in, 5 out]
    }
  }
